vi "Same name VI.vi"(8 "error in (no error)":errorcluster, 9 "Numeric":dbl=4.0, 10 "Numeric 3":dbl, 11 "ChildClass in":refnum<class "ChildClass.lvclass">) -> (0 "error out":errorcluster, 1 "Numeric 2":dbl, 3 "ChildClass out":refnum<class "ChildClass.lvclass">)   [LabVIEW 2022 SP3, in "ChildClass.lvclass"]
uses:
  ChildClass.lvclass
  ChildClass.lvclass/ChildClass.ctl
  BaseClass/BaseClass.lvclass
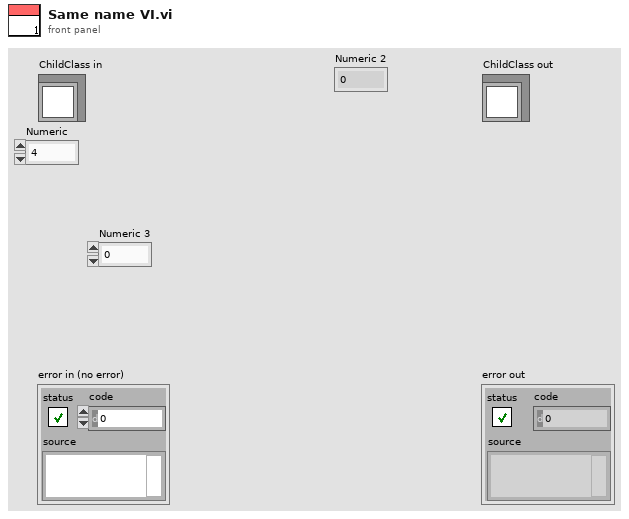
[diagram p1: front panel]
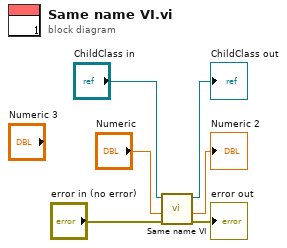
[diagram p0: block diagram]
diagram:
  n1 = call-parent "Same name VI.vi"("error in (no error)"="error in (no error)", "Numeric"="Numeric", "BaseClass in"="ChildClass in") -> ("error out"=→"error out":errorcluster, "Numeric 2"=→"Numeric 2":dbl, "BaseClass out"=→"ChildClass out":refnum<class "ChildClass.lvclass">)  [unwired: 6 in]
